vi "Pockels Cal-Get cal files name.vi"() -> (3 "Filtered Array out":string[](array[string]))   [LabVIEW 2017]
uses:
  Typedefs/Which path.ctl
  <userlib>/_OpenG.lib/array/array.llb/Conditional Auto-Indexing Tunnel (String)__ogtk.vi
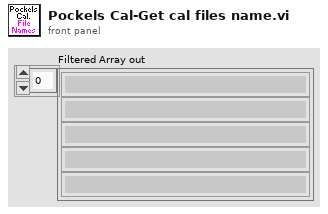
[diagram p1: front panel]
types:
  T1 = typedef "Which path.ctl" = enum16{"Configuration Files", "Calibration Files", "Images", "Setup.ini", "Loaded User profile.ini", "User's-Previous session.ini", "New user profile.ini", "Selected User profile.ini", "User profiles folder", "Power meter scaling.txt", "FOV Cal.ini"}
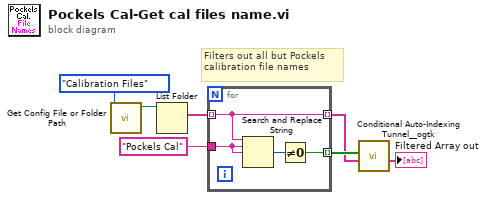
[diagram p0: block diagram]
diagram:
  # "Filters out all but Pockels calibration file names"
  n1 = call "Get Config File or Folder Path.vi"("Which file or folder?"=Which_path."Calibration Files" ("Which path?")) -> ("File Path"=w6:path)  [unwired: 8 in, 2 out]
  n2 = List Folder(path=w6) -> (filenames=w5:string[])  [unwired: 3 in, 3 out]
  n3 = for {
    tunnel: w5 -> [w8] mode=indexing
    tunnel: "Pockels Cal" ("pattern (all files)") -> [w11]
    tunnel: [w9] -> w3 mode=indexing
    tunnel: [w8] -> w2 mode=indexing
    n4 = Search and Replace String(input string=w8, search string=w11, replace string=w11) -> (number of replacements=w10:i32)  [unwired: 5 in, 3 out]
    n5 = Not Equal To 0?(x=w10) -> (x != 0?=w9:bool)
  }
  n6 = call-poly <userlib>:"Conditional Auto-Indexing Tunnel__ogtk.vi"("Array in"=w2, "Elements to keep"=w3) -> ("Filtered Array out"=→"Filtered Array out":string[])  [unwired: 5 in]
